vi "Ortho.vi"(8 "error in (no error)":errorcluster, 10 "boundaries in":T1, 11 "class data in":refnum<class "SceneRoot.lvclass">) -> (0 "error out":errorcluster, 3 "class data out":refnum<class "SceneRoot.lvclass">)   [LabVIEW 2010, in "RenderBase.lvlib" / "SceneRoot.lvclass"]
doc: "Sets up an orthographic projection."
uses:
  SceneRoot.lvclass
  SceneRoot.lvclass/SceneRoot.ctl
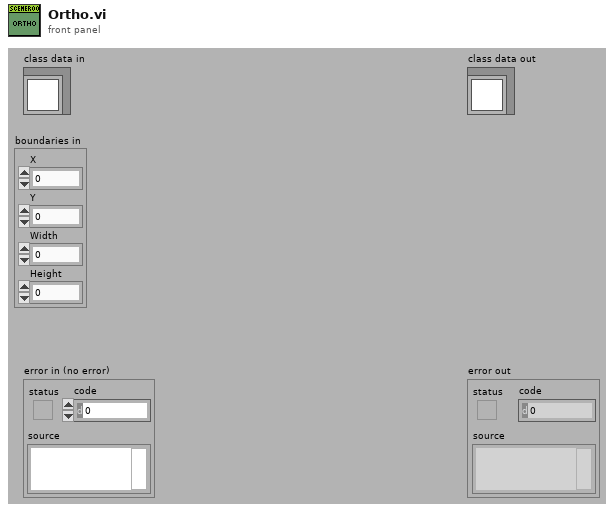
[diagram p1: front panel]
types:
  T1 = cluster{"X":sgl, "Y":sgl, "Width":sgl, "Height":sgl}
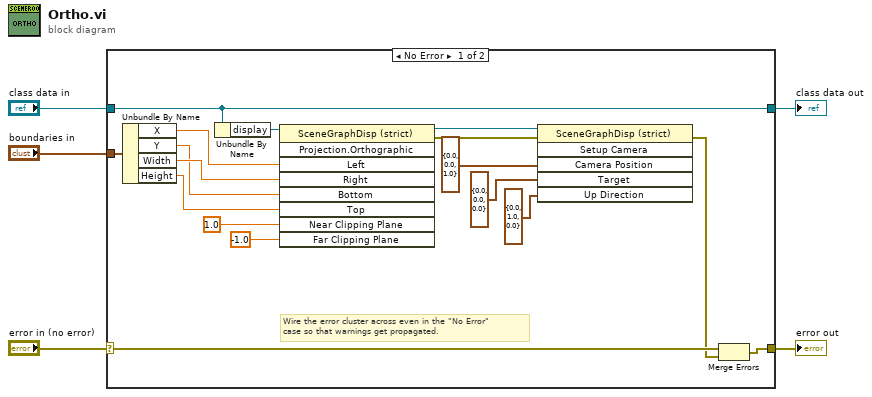
[diagram p0: block diagram]
diagram:
  n1 = case shown="No Error" "error in (no error)" {
    selector: "error in (no error)" -> [w22 w24]
    tunnel: [w7 w24] -> w4
    tunnel: [w10 w23] -> w2
    tunnel: "class data in" -> [w10 w23]
    tunnel: "boundaries in" -> [w21 _]
    frame No Error {
      # "Wire the error cluster across even in the \"No Error\"\ncase so that warnings get propagated."
      n2 = Unbundle By Name(w21) -> ("X"=w15:sgl, "Y"=w13:sgl, "Width"=w14:sgl, "Height"=w12:sgl)
      n3 = Unbundle By Name(w10) -> ("display"=w9:refnum<vi>)
      n4 = invoke on="Invoke Node" class="SceneGraphDisp (strict)" method="Projection.Orthographic"(reference=w9, "Left"=w15, "Right"=w14, "Bottom"=w13, "Top"=w12, "Near Clipping Plane"=sgl 1.0, "Far Clipping Plane"=sgl -1.0) -> (reference out=w11:refnum<vi>, error out=w8:errorcluster)  [unwired: 2 in, 7 out]
      n5 = invoke on="Invoke Node" class="SceneGraphDisp (strict)" method="Setup Camera"(reference=w11, error in=w8, "Camera Position"=cluster{"X":sgl, "Y":sgl, "Z":sgl} {"X"=0.0, "Y"=0.0, "Z"=1.0}, "Target"=cluster{"X":sgl, "Y":sgl, "Z":sgl} {"X"=0.0, "Y"=0.0, "Z"=0.0}, "Up Direction"=cluster{"X":sgl, "Y":sgl, "Z":sgl} {"X"=0.0, "Y"=1.0, "Z"=0.0}) -> (error out=w6:errorcluster)  [unwired: 1 in, 5 out]
      n6 = Merge Errors(w22, w6) -> (w7:errorcluster)
    }
    frame Error {
    }
  }
  "error out" <- w4
  "class data out" <- w2
